vi "GetSessions.vi"(11 "REST Client in":refnum<class "REST Client.lvclass">) -> (3 "Response body":string)   [LabVIEW 2017]
uses:
  <vilib>/addons/_JKI.lib/REST Client/classes/REST Client/REST Client.lvclass
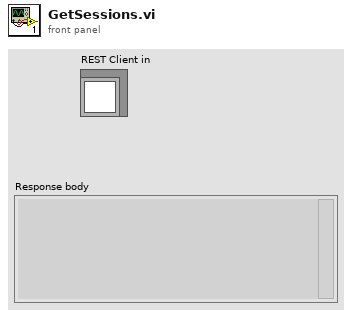
[diagram p1: front panel]
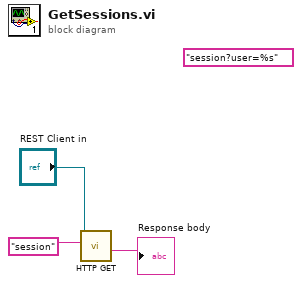
[diagram p0: block diagram]
diagram:
  (unwired) "session?user=%s" ("format string")
  n1 = call-dynamic "HTTP GET.vi"("Path"="session", "REST Client in"="REST Client in") -> ("Response body"=→"Response body":string)  [unwired: 4 in, 5 out]
